vi "PS On.vi"(8 "error in":errorcluster, 11 "SR3XXX in":refnum<class "SR3XXX HVPS.lvclass">) -> (0 "error out":errorcluster, 3 "SR3XXX out":refnum<class "SR3XXX HVPS.lvclass">)   [LabVIEW 2013, in "SR3XXX HVPS.lvclass"]
uses:
  SR3XXX HVPS.lvclass
  Reusable/Session APIs/Serial/Typedefs/Session Handle.ctl
  Reusable/Session APIs/Serial/Serial Session.lvclass
  Base/Session HVPS.lvclass/Session HVPS.ctl
  Base/Read hSession.vi
  Reusable/Session APIs/Serial/Public/Asynchronous Write.vi
  <userlib>/_Session Fwk/Session - Root.lvclass
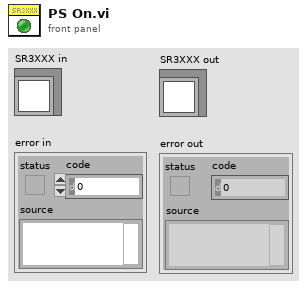
[diagram p1: front panel]
types:
  T1 = typedef "Serial Session.lvclass/Session Handle.ctl" = refnum<data-value>
  T2 = typedef "Session - Root.lvclass/Session Handle.ctl" = refnum<data-value>
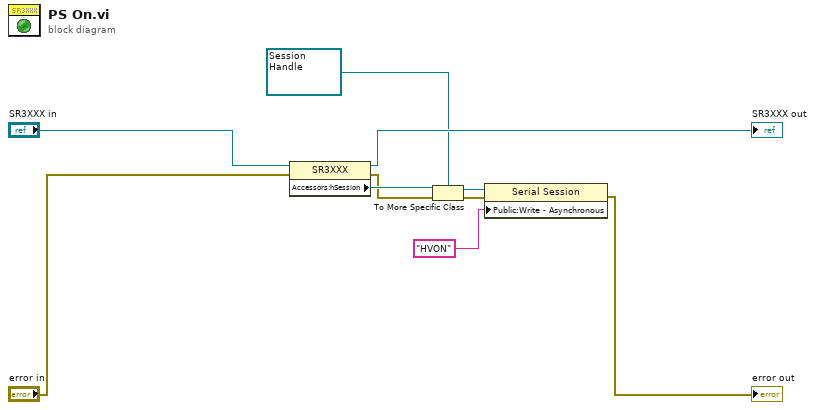
[diagram p0: block diagram]
diagram:
  n1 = property class="SR3XXX"(reference="SR3XXX in", error in="error in") -> (reference out=→"SR3XXX out":refnum<class "SR3XXX HVPS.lvclass">, error out=w2:errorcluster, "Accessors:hSession"=w8:T2)
  n2 = To More Specific Class(target class=T1 refnum ("Session Handle"), reference=w8, error in=w2) -> (specific class reference=w6:T1, error out=w5:errorcluster)
  n3 = property class="Serial Session"(reference=w6, error in=w5, "Public:Write - Asynchronous"="HVON" ("Cmd")) -> (error out=→"error out":errorcluster)  [unwired: 1 out]
